vi "Read Response ADC.vi"(8 "error in (no error)":errorcluster, 11 "Arduino in":refnum<class "Arduino.lvclass">) -> (0 "error out":errorcluster, 2 "Respuesta":string, 3 "Arduino out":refnum<class "Arduino.lvclass">)   [LabVIEW 2020, in "Arduino.lvclass"]
uses:
  Arduino.lvclass
  Abstracts/Serial Device/Serial Device.lvclass
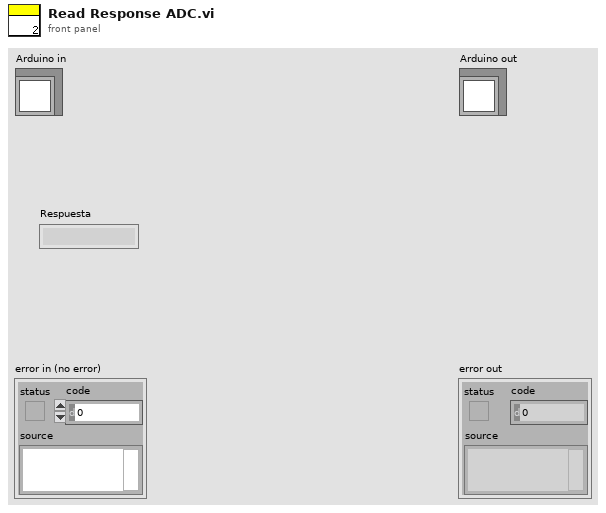
[diagram p1: front panel]
types:
  T1 = typedef "Serial Device.lvclass/serial device brand.ctl" = string
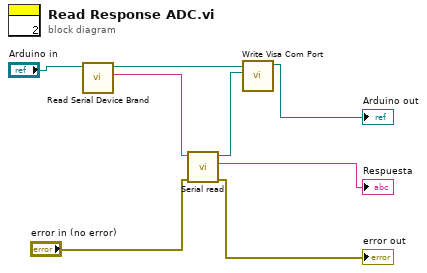
[diagram p0: block diagram]
diagram:
  n1 = call-dynamic "Read Serial Device Brand.vi"("Serial Device in"="Arduino in") -> ("Serial Device Brand"=w8:T1, "Serial Device out"=w3:refnum<class "Arduino.lvclass">)  [unwired: 8 in, 1 out]
  n2 = call "Serial read.vi"("error in (no error)"="error in (no error)", "VISA resource name in"=w8) -> ("error out"=→"error out":errorcluster, "Respuesta"=→"Respuesta":string, "VISA resource name out"=w1:refnum<visa-resource-name>)  [unwired: 7 in]
  n3 = call-dynamic "Write Visa Com Port.vi"("Visa Com Port"=w1, "Serial Device in"=w3) -> ("Serial Device out"=→"Arduino out":refnum<class "Arduino.lvclass">)  [unwired: 8 in, 1 out]
